vi "MT Measure Offset PSK Quadrature Impairments.vi"(0 "recovered complex waveform":T7={"t0"=0.0, "dt"=1.0, "Y"=[]} {"Y" format="%.3f"; "dt" format="%^.2e"; "t0" format="%.4f"}, 1 "input bit stream":i8[](array[numeric]), 3 "impairment measurement window":T4={"start index (symbols)"=0, "width (symbols) (-1: all)"=-1}, 4 "Reference Filter":dbl[](array[numeric]), 5 "error in (no error)":errorcluster, 6 "Offset PSK System Parameters":T3={"samples per symbol (16)"=16, "symbol map"=[], "differential Offset PSK"=enum."disable"} {"symbol map" format="%.3f"}, 7 "impairment definition":enum16{"Vertical Shear", "Axis Shear"}(ring), 11 "reset? (T)":bool=TRUE) -> (10 "magnitude error":T2 {"individual symbol measurements (%)" format="%.2f"; "peak measurement (%)" format="%.2f"; "RMS measurement (%)" format="%.2f"}, 12 "DC offset measurements":T5 {"origin offset (dB)" format="%.2f"; "Q (%)" format="%.2f"; "I (%)" format="%.2f"}, 13 "quadrature skew (deg)":dbl format="%.2f", 14 "IQ gain imbalance (dB)":dbl format="%.2f", 15 "phase error":T6 {"individual symbol measurements (deg)" format="%.2f"; "peak measurement (deg)" format="%.2f"; "RMS measurement (deg)" format="%.2f"}, 16 "Offset EVM":T2 {"individual symbol measurements (%)" format="%.2f"; "peak measurement (%)" format="%.2f"; "RMS measurement (%)" format="%.2f"}, 17 "EVM":T1 {"RMS measurement, %" format="%#_2f"}, 18 "modulation error ratio (dB)":dbl format="%.2f", 19 "error out":errorcluster)   [LabVIEW 2020, in "niDMT.lvlib"]
doc: "Measures and reports quadrature impairments over a single user-specified window. This VI must be called once for each measurement window. \n\nThis polymorphic instance calculates and reports offset PSK quadrature impairments on a symbol-by-symbol basis at the symbol timing."
uses:
  <vilib>/addons/Modulation/niDMT.lvlib
  <vilib>/addons/Modulation/Analog/controls/Complex Data Waveform.ctl
  <vilib>/addons/Modulation/Digital/Support/Controls/Offset PSK System Parameters.ctl
  <vilib>/addons/Modulation/niAMT.lvlib
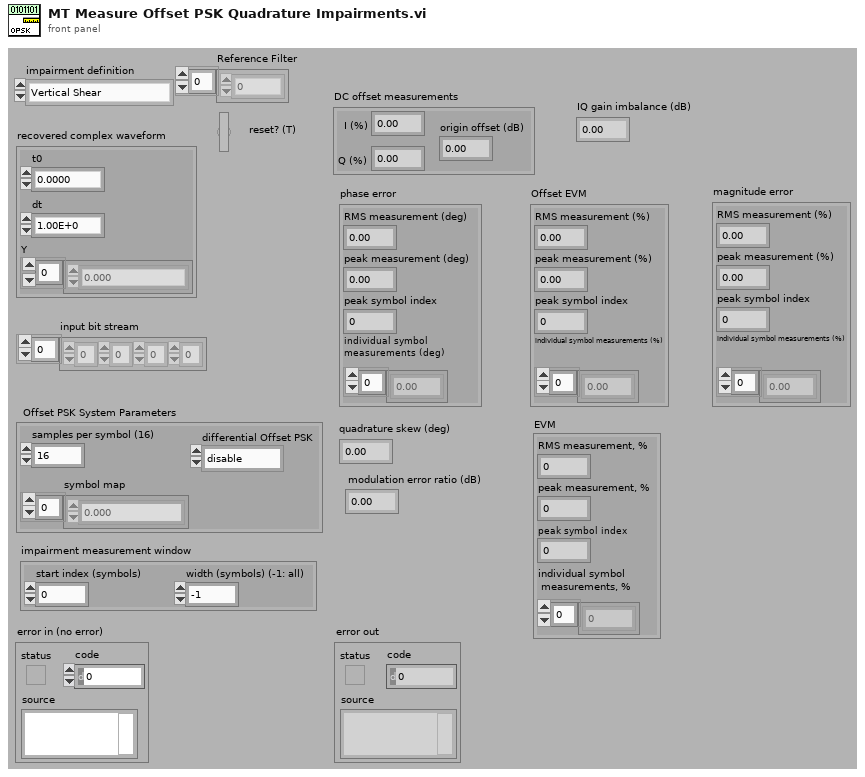
[diagram p1: front panel]
types:
  T1 = cluster{"RMS measurement, %":dbl, "peak measurement, %":dbl, "peak symbol index":i32, "individual symbol\n measurements, %":dbl[]}
  T2 = cluster{"RMS measurement (%)":dbl, "peak measurement (%)":dbl, "peak symbol index":i32, "individual symbol measurements (%)":dbl[]}
  T3 = typedef "niDMT.lvlib/Offset PSK System Parameters.ctl" = cluster{"samples per symbol (16)":i32, "symbol map":cdb[], "differential Offset PSK":enum16{"disable", "enable"}}
  T4 = cluster{"start index (symbols)":i32, "width (symbols) (-1: all)":i32}
  T5 = cluster{"I (%)":dbl, "Q (%)":dbl, "origin offset (dB)":dbl}
  T6 = cluster{"RMS measurement (deg)":dbl, "peak measurement (deg)":dbl, "peak symbol index":i32, "individual symbol measurements (deg)":dbl[]}
  T7 = typedef "niAMT.lvlib/Complex Data Waveform.ctl" = cluster{"t0":dbl, "dt":dbl, "Y":cdb[]}
  T8 = enum16{"FSK", "PSK", "QAM", "MSK", "PAM", "ASK", "CPM"}
  T9 = cluster{"RMS Measurement, %":dbl, "Peak Measurement, %":dbl, "Peak Symbol Index":i32, "Individual Symbol Measurements, %":dbl[]}
  T10 = cluster{"I, %":dbl, "Q, %":dbl, "Origin Offset, dB":dbl}
  T11 = cluster{"RMS Measurement, deg":dbl, "Peak Measurement, deg":dbl, "Peak Symbol Index":i32, "Individual Symbol Measurements, deg":dbl[]}
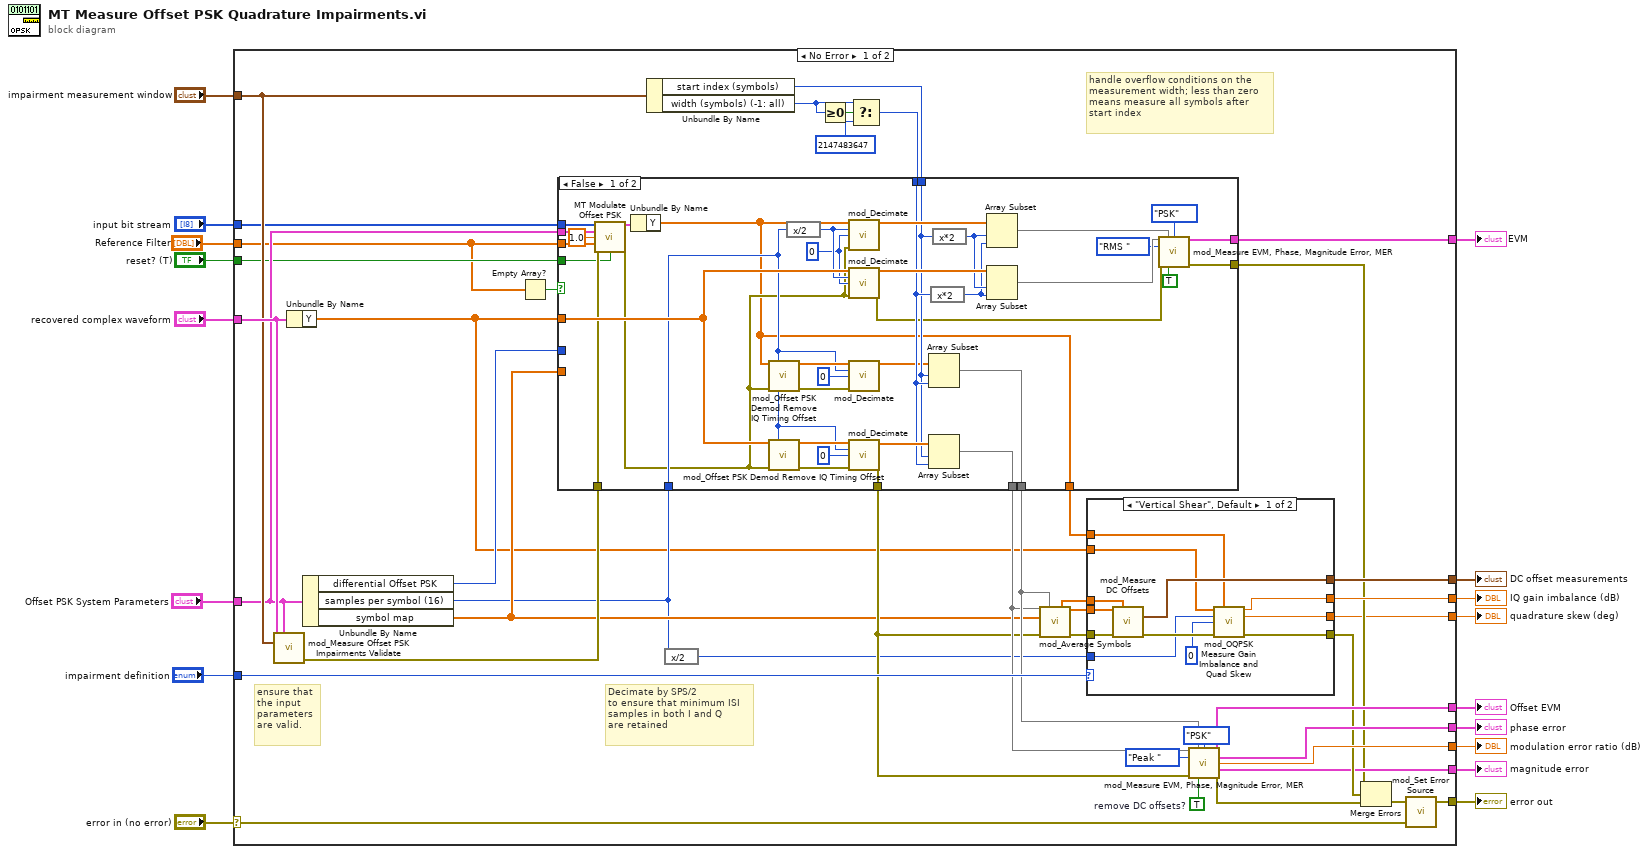
[diagram p0: block diagram]
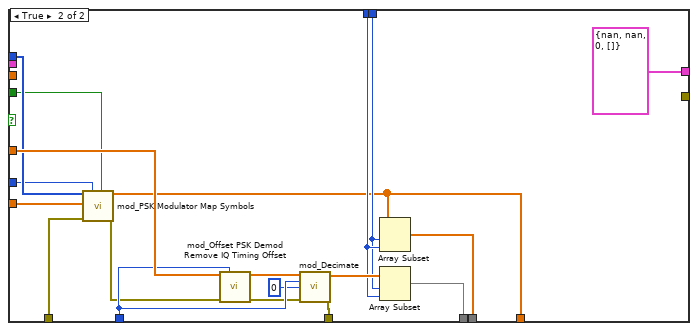
[diagram p2: hidden frame]
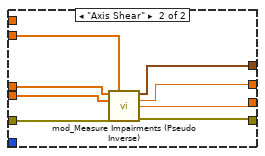
[diagram p3: hidden frame]
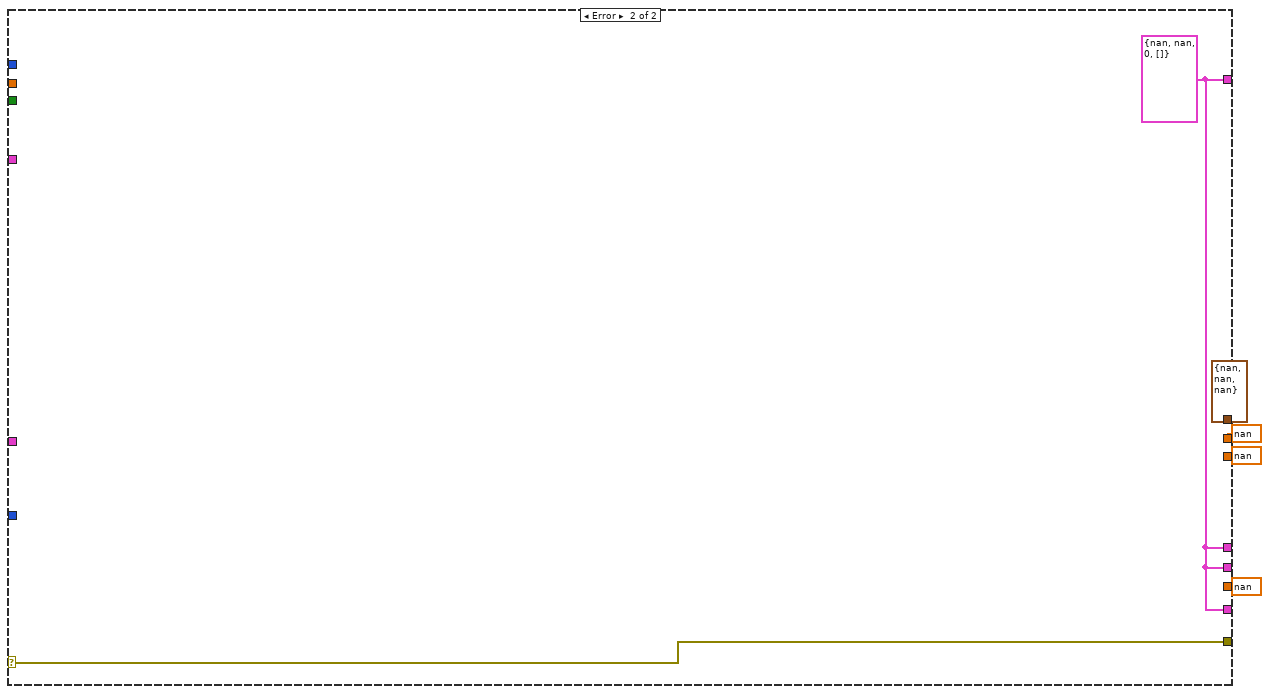
[diagram p4: hidden frame]
diagram:
  n1 = case shown="No Error" "error in (no error)" {
    selector: "error in (no error)" -> [w52 w143]
    tunnel: "recovered complex waveform" -> [w58 _]
    tunnel: [w54 T10 {"I, %"=nan, "Q, %"=nan, "Origin Offset, dB"=nan} ("DC Offset Measurements")] -> w7
    tunnel: [w56 w139] -> w15
    tunnel: [w60 w139] -> w14
    tunnel: [w49 nan ("IQ gain imbalance (dB)")] -> w13
    tunnel: [w51 w143] -> w12
    tunnel: "input bit stream" -> [w29 _]
    tunnel: "impairment measurement window" -> [w57 _]
    tunnel: [w55 nan ("Modulation Error Ratio, dB")] -> w9
    tunnel: [w23 nan ("quadrature skew (deg)")] -> w8
    tunnel: "Offset PSK System Parameters" -> [w36 _]
    tunnel: "reset? (T)" -> [w28 _]
    tunnel: [w42 w139] -> w4
    tunnel: "impairment definition" -> [w41 _]
    tunnel: "Reference Filter" -> [w22 _]
    tunnel: [w37 w139] -> w1
    frame No Error {
      w45 = TRUE  # remove DC offsets?
      # "Decimate by SPS/2\nto ensure that minimum ISI\nsamples in both I and Q\nare retained"
      # "ensure that \nthe input \nparameters \nare valid."
      # "handle overflow conditions on the\nmeasurement width; less than zero\nmeans measure all symbols after\nstart index"
      n2 = call <vilib>:"mod_Measure Offset PSK Impairments Validate.vi"("Input Complex Waveform"=w58, "PSK System Parameters"=w36, "Impairment Measurement Window"=w57) -> ("error out"=w30:errorcluster)  [unwired: 12 out]
      n3 = Unbundle By Name(w58) -> ("Y"=w19:cdb[])
      n4 = Unbundle By Name(w36) -> ("differential Offset PSK"=w26:enum16{"disable", "enable"}, "samples per symbol (16)"=w21:i32, "symbol map"=w25:cdb[])
      n5 = Empty Array?(array=w22) -> (empty?=w27:bool)
      n6 = Unbundle By Name(w57) -> ("start index (symbols)"=w35:i32, "width (symbols) (-1: all)"=w43:i32)
      n7 = expression code="x/2"(w21) -> (w20:i32)
      n8 = Greater Or Equal To 0?(x=w43) -> (x >= 0?=w44:bool)
      n9 = Select(t=w43, s=w44, f=2147483647) -> (s? t:f=w38:i32)
      n10 = case shown="False" w27 {
        tunnel: w19 -> [w96 w117]
        tunnel: w38 -> [w90 w114]
        tunnel: [w88 T9 {"RMS Measurement, %"=nan, "Peak Measurement, %"=nan, "Peak Symbol Index"=0, "Individual Symbol Measurements, %"=[]} ("EVM")] -> w37
        tunnel: w36 -> [w87 _]
        tunnel: w22 -> [w86 _]
        tunnel: w35 -> [w83 w113]
        tunnel: w21 -> [w63 w112]
        tunnel: [w81 w111] -> w34
        tunnel: [w78 w110] -> w33
        tunnel: [w77 w109] -> w32
        tunnel: [w74 _] -> w24
        tunnel: w30 -> [w71 w106]
        tunnel: w29 -> [w70 w105]
        tunnel: w28 -> [w69 w102]
        tunnel: w26 -> [_ w104]
        tunnel: w25 -> [_ w103]
        tunnel: [w61 w99] -> w18
        frame False {
          w82 = 0 ("Offset")
          n11 = call <vilib>:"MT Modulate Offset PSK.vi"("input bit stream"=w70, "Offset PSK system parameters"=w87, "symbol rate (Hz)"=1.0, "pulse shaping filter coefficients"=w86, "error in (no error)"=w71, "reset? (T)"=w69) -> ("output complex waveform"=w85:T7, "error out"=w62:errorcluster)  [unwired: 1 in, 7 out]
          n12 = Unbundle By Name(w85) -> ("Y"=w61:cdb[])
          n13 = call <vilib>:"mod_Offset PSK Demod Remove IQ Timing Offset.vi"("Signal In"=w61, "Samples Per Symbol"=w63, "error in (no error)"=w62) -> ("Un-offset Signal"=w65:cdb[], "error out"=w66:errorcluster)  [unwired: 2 in, 9 out]
          n14 = call <vilib>:"mod_Offset PSK Demod Remove IQ Timing Offset.vi"("Signal In"=w96, "Samples Per Symbol"=w63, "error in (no error)"=w62) -> ("Un-offset Signal"=w94:cdb[], "error out"=w76:errorcluster)  [unwired: 2 in, 9 out]
          n15 = expression code="x/2"(w63) -> (w84:i32)
          n16 = call <vilib>:"mod_Decimate.vi"("Signal In"=w61, "Samples Per Symbol (16)"=w84, "Offset"=w82, "error in (no error)"=w62) -> ("Signal Out"=w95:cdb[])  [unwired: 1 in, 10 out]
          n17 = call <vilib>:"mod_Decimate.vi"("Signal In"=w96, "Samples Per Symbol (16)"=w84, "Offset"=w82, "error in (no error)"=w62) -> ("Signal Out"=w98:cdb[], "error out"=w68:errorcluster)  [unwired: 1 in, 9 out]
          n18 = call <vilib>:"mod_Decimate.vi"("Signal In"=w65, "Samples Per Symbol (16)"=w63, "Offset"=0, "error in (no error)"=w66) -> ("Signal Out"=w64:cdb[])  [unwired: 1 in, 10 out]
          n19 = call <vilib>:"mod_Decimate.vi"("Signal In"=w94, "Samples Per Symbol (16)"=w63, "Offset"=0, "error in (no error)"=w76) -> ("Signal Out"=w93:cdb[], "error out"=w77:errorcluster)  [unwired: 1 in, 9 out]
          n20 = Array Subset(array=w64, index=w83, length=w90) -> (w81:cdb[])
          n21 = Array Subset(array=w93, index=w83, length=w90) -> (w78:cdb[])
          n22 = expression code="x*2"(w90) -> (w89:i32)
          n23 = expression code="x*2"(w83) -> (w92:i32)
          n24 = Array Subset(array=w95, index=w92, length=w89) -> (w80:cdb[])
          n25 = Array Subset(array=w98, index=w92, length=w89) -> (w79:cdb[])
          n26 = call <vilib>:"mod_Measure EVM, Phase, Magnitude Error, MER.vi"("Recovered Signal"=w79, "Detected Signal"=w80, "EVM Normalization Type"=enum16{"Peak ", "RMS "}."RMS ", "error in (no error)"=w68, "remove DC offsets? (T)"=TRUE, "Modulation Type"=T8."PSK") -> ("EVM"=w88:T9, "error out"=w74:errorcluster)  [unwired: 8 out]
        }
        frame True {
          n27 = call <vilib>:"mod_PSK Modulator Map Symbols.vi"("Input Bit Stream"=w105, "Differential PSK Enable (disable)"=w104, "Symbol Map"=w103, "error in (no error)"=w106, "Reset? (T)"=w102) -> ("Symbols"=w99:cdb[], "error out"=w100:errorcluster)  [unwired: 2 in, 7 out]
          n28 = call <vilib>:"mod_Offset PSK Demod Remove IQ Timing Offset.vi"("Signal In"=w117, "Samples Per Symbol"=w112, "error in (no error)"=w100) -> ("Un-offset Signal"=w116:cdb[], "error out"=w108:errorcluster)  [unwired: 2 in, 9 out]
          n29 = call <vilib>:"mod_Decimate.vi"("Signal In"=w116, "Samples Per Symbol (16)"=w112, "Offset"=0, "error in (no error)"=w108) -> ("Signal Out"=w115:cdb[], "error out"=w109:errorcluster)  [unwired: 1 in, 9 out]
          n30 = Array Subset(array=w99, index=w113, length=w114) -> (w111:cdb[])
          n31 = Array Subset(array=w115, index=w113, length=w114) -> (w110:cdb[])
        }
      }
      n32 = call <vilib>:"mod_Average Symbols.vi"("Recovered Symbols"=w33, "Detected Symbols"=w34, "Symbol Map"=w25, "error in (no error)"=w32) -> ("Grouped Detected Symbols"=w47:cdb[], "Averaged Symbols"=w46:cdb[], "error out"=w48:errorcluster)  [unwired: 9 out]
      n33 = case shown="\"Vertical Shear\", Default" w41 {
        tunnel: [w129 w134] -> w54
        tunnel: [w124 w135] -> w50
        tunnel: [w122 w133] -> w49
        tunnel: w48 -> [w126 w136]
        tunnel: w47 -> [w128 w137]
        tunnel: w46 -> [w127 w132]
        tunnel: w19 -> [w123 w131]
        tunnel: [w121 w130] -> w23
        tunnel: w20 -> [w120 _]
        tunnel: w18 -> [w118 _]
        frame "Vertical Shear", Default {
          n34 = call <vilib>:"mod_Measure DC Offsets.vi"("Averaged Symbols"=w127, "Grouped Detected Symbols"=w128, "error in (no error)"=w126) -> ("DC Offset Measurements"=w129:T10, "error out"=w125:errorcluster)  [unwired: 1 in, 10 out]
          n35 = call <vilib>:"mod_OQPSK Measure Gain Imbalance and Quad Skew.vi"("Recovered Symbols"=w123, "Detected Symbols"=w118, "Decimation Factor"=w120, "Offset"=0, "error in (no error)"=w125) -> ("IQ Gain Imbalance, dB"=w122:dbl, "Quadrature Skew, deg"=w121:dbl, "error out"=w124:errorcluster)  [unwired: 8 in]
        }
        frame "Axis Shear" {
          n36 = call <vilib>:"mod_Measure Impairments (Pseudo Inverse).vi"("Grouped detected symbols"=w137, "Recovered Complex Waveform"=w131, "Averaged symbols"=w132, "error in (no error)"=w136) -> ("DC Offset Measurements"=w134:T10, "IQ gain imbalance (dB)"=w133:dbl, "quadrature skew (deg)"=w130:dbl, "error out"=w135:errorcluster)  [unwired: 8 out]
        }
      }
      n37 = call <vilib>:"mod_Measure EVM, Phase, Magnitude Error, MER.vi"("Recovered Signal"=w33, "Detected Signal"=w34, "EVM Normalization Type"=enum16{"Peak ", "RMS "}."Peak ", "error in (no error)"=w32, "remove DC offsets? (T)"=w45, "Modulation Type"=T8."PSK") -> ("EVM"=w60:T9, "Phase Error"=w56:T11, "Modulation Error Ratio, dB"=w55:dbl, "magnitude error"=w42:T9, "error out"=w59:errorcluster)  [unwired: 5 out]
      n38 = Merge Errors(w24, w50, w59) -> (w53:errorcluster)
      n39 = call <vilib>:"mod_Set Error Source.vi"("initial error in (no error)"=w52, "final error in (no error)"=w53) -> ("error out"=w51:errorcluster)  [unwired: 3 in]
    }
    frame Error {
      w139 = T9 {"RMS Measurement, %"=nan, "Peak Measurement, %"=nan, "Peak Symbol Index"=0, "Individual Symbol Measurements, %"=[]} ("EVM")
    }
  }
  "error out" <- w12
  "IQ gain imbalance (dB)" <- w13
  "quadrature skew (deg)" <- w8
  "phase error" <- w15
  "Offset EVM" <- w14
  "modulation error ratio (dB)" <- w9
  "DC offset measurements" <- w7
  "magnitude error" <- w4
  "EVM" <- w1
